vi "Create GB (2).vi"(5 "Max # of atoms":i32=9999999, 6 "Edge Duplication Range":dbl=3.0, 7 "Skip cleanup if no subset":bool=TRUE, 8 "Reduce to Repeating":T3={"Slab X"=4.6, "Slab Y"=4.0, "Tolerance (A)"=0.5, "Presorted?"=FALSE}, 9 "Min Seperation Distance (A)":dbl=2.0, 10 "Grain Growth and Geometry":T4={"Min Grain 1 Length (A)"=6.0, "Min Grain 2 Length (A)"=6.0, "Max Grain Height (A)"=90.0, "Max Grain Width (A)"=90.0, "Grain 1 Start"=-0.001, "Overlap Region (A)"=0.001}, 11 "Grain Boundary Definition":T5={"Grain 1 Orientation"=[1.0, 0.6019417241891012, 0.029651947654046266], "Grain 2 Orientation"=[1.0, 0.730727623275494, 0.2205637301176], "Twist Angle (Deg)"=0.0, "Translation Vector"=[0.0, 0.0, 0.0]}) -> (0 "GB Data":string[][](array[string])=[["Grain 1, h", "Grain 1, k", "Grain 1, L", "Grain 2, h", "Grain 2, k", "Grain 2, L", "Twist Angle (Deg)", "Translation Tx", "Translation Ty", "Translation Tz", "Tilt Angle (Deg)", "Viewing Angle, h", "Viewing Angle, k", "Viewing Angle, L", "Grain 1 Length (factor)", "Grain 2 Length (factor", "Max Grain Height (A)", "Max Grain Width (A)", "Grain 1 Start", "Overlap Region (A)", "Reduction Slab X", "Reduction Slab Y", "Reduction Tolerance (A)", "Min Atomic Separation Distance", "Edge Duplication Range", "# Atoms"], ["1.000000", "0.601942", "0.029652", "1.000000", "0.730728", "0.220564", "0.000000", "0.000000", "0.000000", "0.000000", "10.024930", "1.000000", "-1.661290", "0.000000", "1.000000", "1.000000", "90.000000", "90.000000", "-0.001000", "0.001000", "4.600000", "4.000000", "0.500000", "2.000000", "3.000000", "12135.000000"]], 1 "Reduced Orthorhombic?":bool, 2 "Reduced Rhombahedral?":bool, 3 "Grain Boundary":T6={"Structure Name"="(0.00) twist [1.000,0.602,0.030] [1.000,0.731,0.221] (0.00,0.00,0.00)T GB", "Lattice vector a"=[270.03, 0.0, 0.0], "Lattice vector b"=[0.0, 270.03, 0.0], "Lattice vector c"=[0.0, 0.0, 6.006], "Atoms Array"=[{"Atom Name"="Cd", "Positions (Direct)"=array6055x3[18165 elements], "Positions (Cartesian)"=array6055x3[18165 elements]}, {"Atom Name"="Te", "Positions (Direct)"=array6080x3[18240 elements], "Positions (Cartesian)"=array6080x3[18240 elements]}], "# of atoms"=12135} {"Atoms Array"."Positions (Cartesian)" format="%#_4f"; "Atoms Array"."Positions (Direct)" format="%#_4f"}, 4 "Ortho and Rhom":T1(array[cluster]) {"Atoms Array"."Positions (Cartesian)" format="%#_4f"; "Atoms Array"."Positions (Direct)" format="%#_4f"})   [LabVIEW 2010]
uses:
  <vilib>/Analysis/NI_AALPro.lvlib
  <vilib>/Analysis/_algsub.llb/Real Vector Norm.vi
  <vilib>/Analysis/NI_AALBase.lvlib
  <vilib>/Analysis/baseanly.llb/A x Vector.vi
  <vilib>/Analysis/baseanly.llb/Real A x B.vi
panel:
  in  "Min Wedge Thickness (A)":dbl=5.0
  out "error out":errorcluster
  out "Original # of atoms":i32=12135
  out "Expected # of Atoms":i32=166
  in  "Integer Tolerance":dbl=0.01
  in  "Predict Best Size":bool
  out "Creation Time":T2={"Time to create primitives"=0, "Time to Grow to Box"=4152, "Time to find subset"=1109, "Time to Cleanup"=1}
  in  "Headers":string[](array[string])=["Grain 1, h", "Grain 1, k", "Grain 1, L", "Grain 2, h", "Grain 2, k", "Grain 2, L", "Twist Angle (Deg)", "Translation Tx", "Translation Ty", "Translation Tz", "Tilt Angle (Deg)", "Viewing Angle, h", "Viewing Angle, k", "Viewing Angle, L", "Grain 1 Length (factor)", "Grain 2 Length (factor", "Max Grain Height (A)", "Max Grain Width (A)", "Grain 1 Start", "Overlap Region (A)", "Reduction Slab X", "Reduction Slab Y", "Reduction Tolerance (A)", "Min Atomic Separation Distance", "Edge Duplication Range", "# Atoms"]
  out "Rhombehedral Atoms":i32=12135
  out "Orthorhombic atoms":i32=12135
  out "Time to Cleanup":u32=1
  out "Time to find subset":u32=1109
  out "Time to Grow to Box":u32=4152
  out "Time to create primitives":u32
  out "Tilt Angle":dbl=10.024929742348679
  out "# of Atoms Removed":i32=28
  out "Repeating Y Length Scale":dbl=13.227303403298492
  out "Repeating X Length Scale":dbl
  out "Mutual Viewing Angle":dbl[](array[numeric])=[1.0, -1.6612903871170226, 0.0]
  in  "Conventional Unit Cell":T6={"Structure Name"="CdTe", "Lattice vector a"=[6.615785553057252, 0.0, 0.0], "Lattice vector b"=[0.0, 6.615785553057252, 0.0], "Lattice vector c"=[0.0, 0.0, 6.615785553057252], "Atoms Array"=[{"Atom Name"="Cd", "Positions (Direct)"=[[0.0, 0.0, 0.0], [0.0, 0.5, 0.5], [0.5, 0.0, 0.5], [0.5, 0.5, 0.0]], "Positions (Cartesian)"=[[0.0, 0.0, 0.0], [0.0, 3.307892776528626, 3.307892776528626], [3.307892776528626, 0.0, 3.307892776528626], [3.307892776528626, 3.307892776528626, 0.0]]}, {"Atom Name"="Te", "Positions (Direct)"=[[0.25, 0.25, 0.25], [0.75, 0.75, 0.25], [0.75, 0.25, 0.75], [0.25, 0.75, 0.75]], "Positions (Cartesian)"=[[1.653946388264313, 1.653946388264313, 1.653946388264313], [4.96183916479294, 4.96183916479294, 1.653946388264313], [4.96183916479294, 1.653946388264313, 4.96183916479294], [1.653946388264313, 4.96183916479294, 4.96183916479294]]}], "# of atoms"=8}
  # "Primitives"
  # "Grain Growth"
  # "Make into repeating cell"
  # "Remove Collisions"
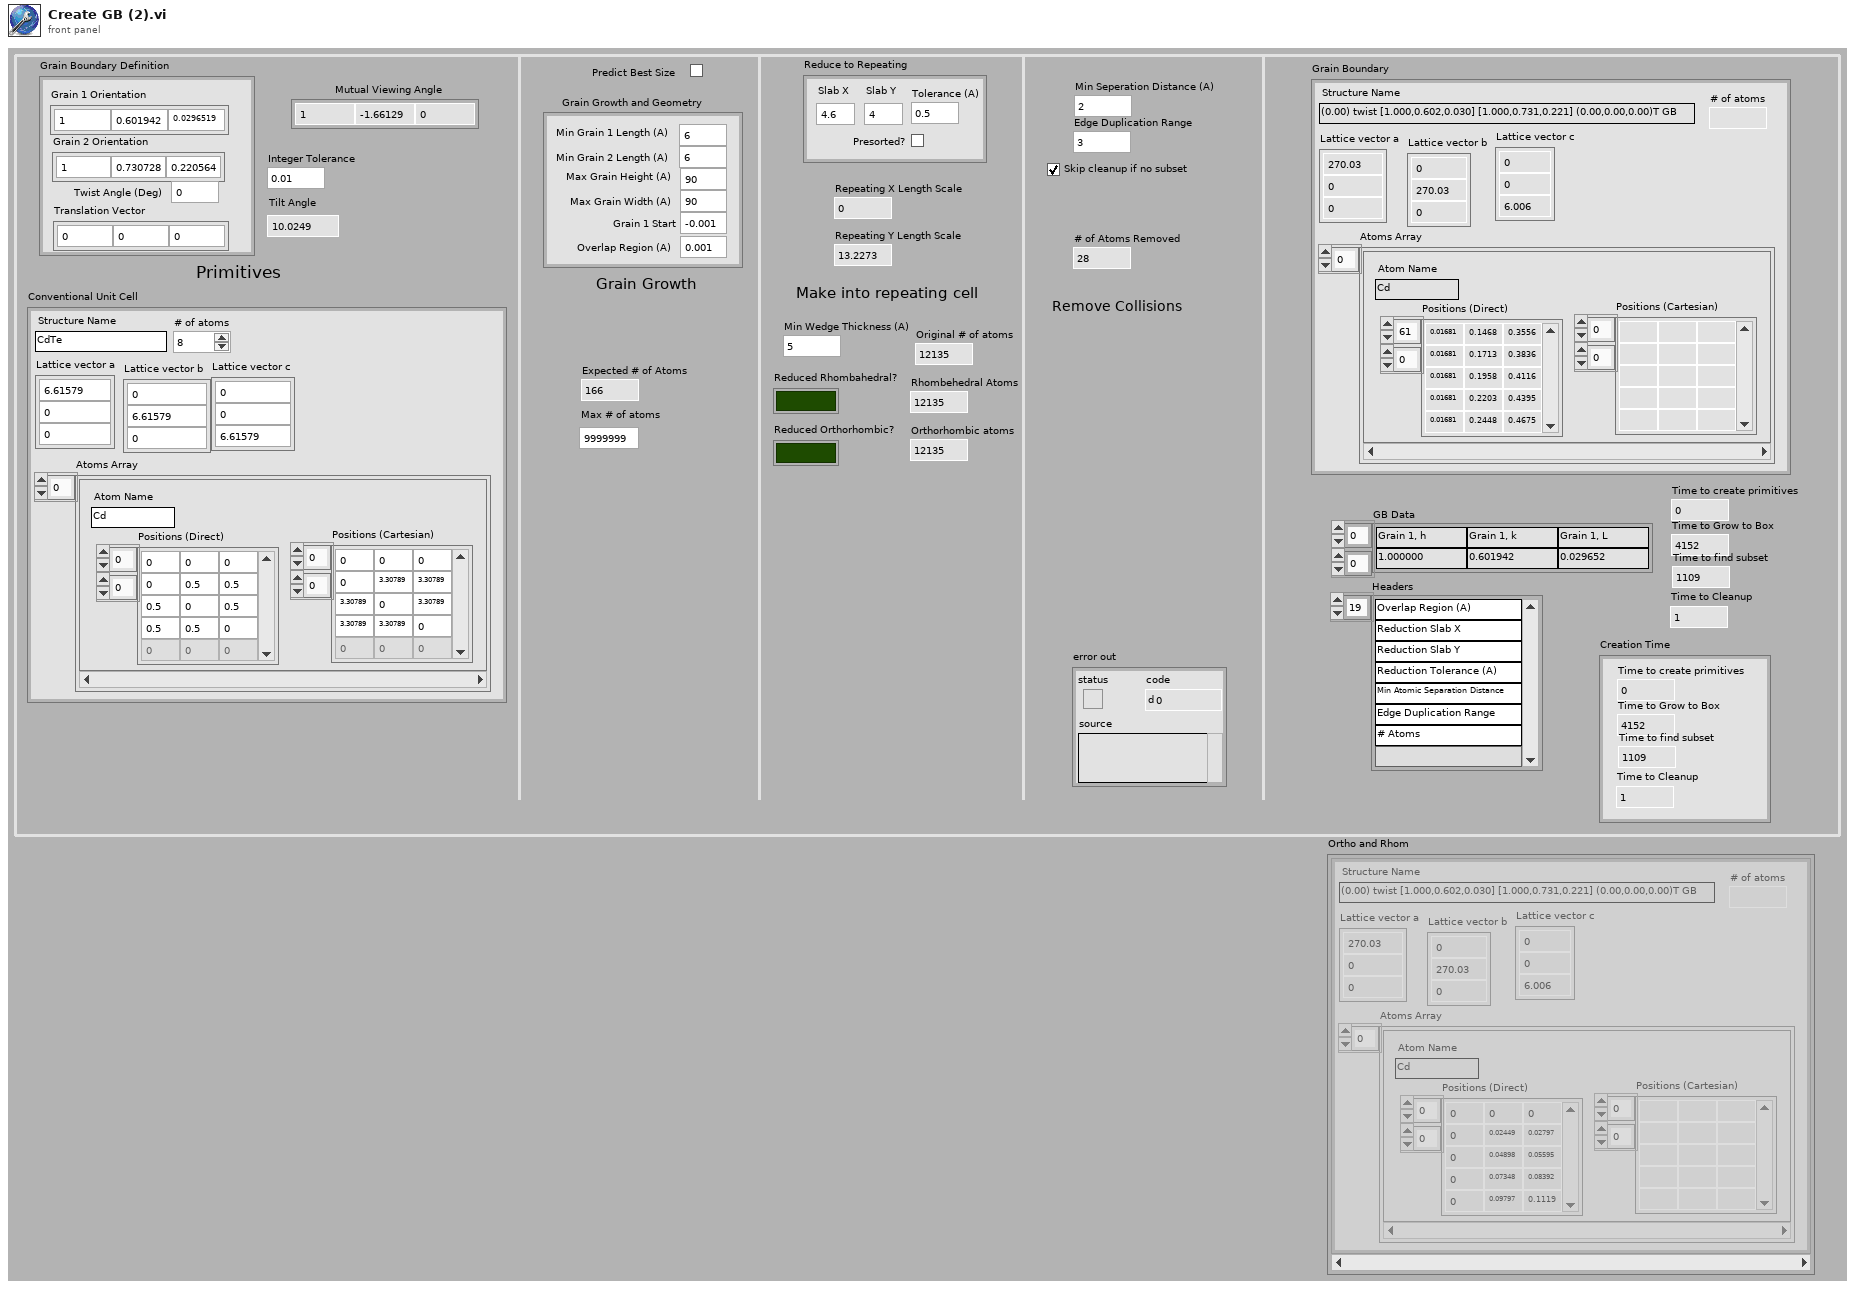
[diagram p1: front panel]
types:
  T1 = cluster{"Structure Name":string, "Lattice vector a":dbl[], "Lattice vector b":dbl[], "Lattice vector c":dbl[], "Atoms Array":cluster{"Atom Name":string, "Positions (Direct)":dbl[][], "Positions (Cartesian)":dbl[][]}[], "# of atoms":i32}[]
  T2 = cluster{"Time to create primitives":u32, "Time to Grow to Box":u32, "Time to find subset":u32, "Time to Cleanup":u32}
  T3 = cluster{"Slab X":dbl, "Slab Y":dbl, "Tolerance (A)":dbl, "Presorted?":bool}
  T4 = cluster{"Min Grain 1 Length (A)":dbl, "Min Grain 2 Length (A)":dbl, "Max Grain Height (A)":dbl, "Max Grain Width (A)":dbl, "Grain 1 Start":dbl, "Overlap Region (A)":dbl}
  T5 = cluster{"Grain 1 Orientation":dbl[], "Grain 2 Orientation":dbl[], "Twist Angle (Deg)":dbl, "Translation Vector":dbl[]}
  T6 = cluster{"Structure Name":string, "Lattice vector a":dbl[], "Lattice vector b":dbl[], "Lattice vector c":dbl[], "Atoms Array":cluster{"Atom Name":string, "Positions (Direct)":dbl[][], "Positions (Cartesian)":dbl[][]}[], "# of atoms":i32}
  T7 = cluster{"Grain 1 Orientation":dbl[], "Grain 2 Orientation":dbl[], "Twist Angle (Deg)":dbl}
  T8 = typedef "NI_Matrix.lvlib/RealMatrix.ctl" = dbl[][]
  T9 = cluster{"Z Min":dbl, "Max Grain Width (A)":dbl, "Z Min":dbl, "Max Grain Height (A)":dbl, "Grain 1 Start":dbl, "# of Atoms":i32}
  T10 = cluster{"Z Min":dbl, "Max Grain Width (A)":dbl, "Z Min":dbl, "Max Grain Height (A)":dbl, dbl, void}
  T11 = cluster{"X Min":dbl, "X Max":dbl, "Y Min":dbl, "Y Max":dbl, "Z Min":dbl, "Z Max":dbl}
  T12 = cluster{"Z Min":dbl, void, "Z Min":dbl, void, "Grain 1 Start":dbl, void}
  T13 = cluster{"Z Min":dbl, void, "Z Min":dbl, void, "Grain 1 Start":dbl, "# of Atoms":i32}
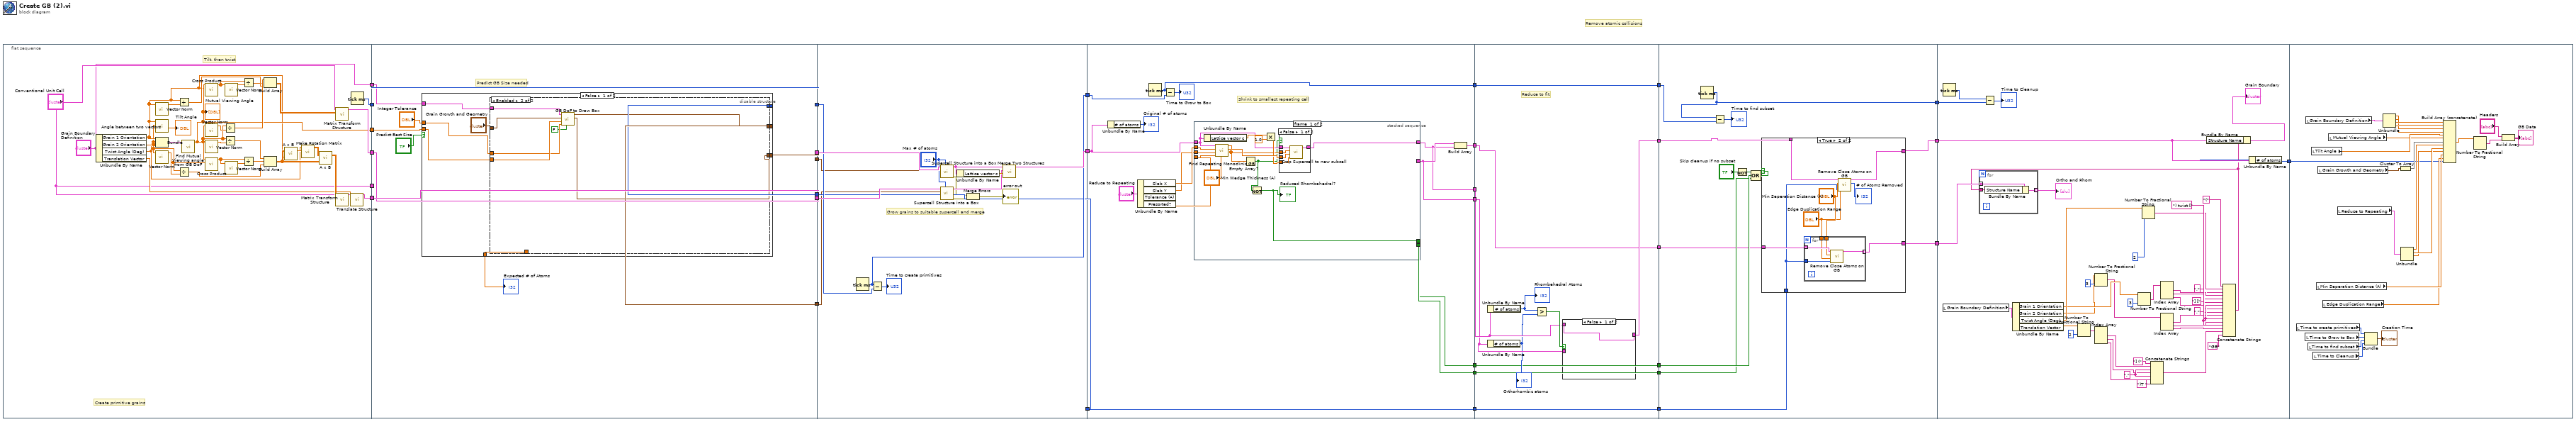
[diagram p0: block diagram]
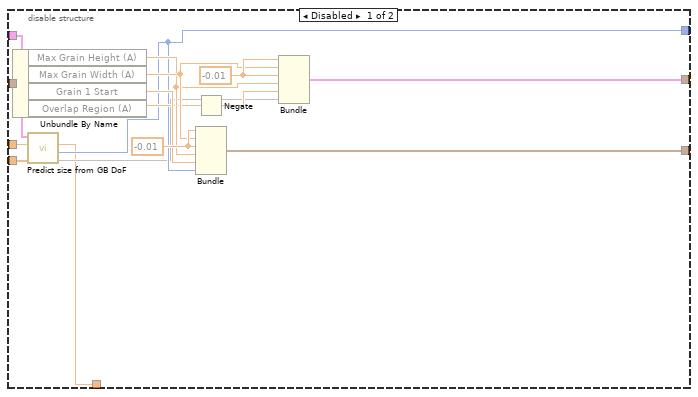
[diagram p2: hidden frame]
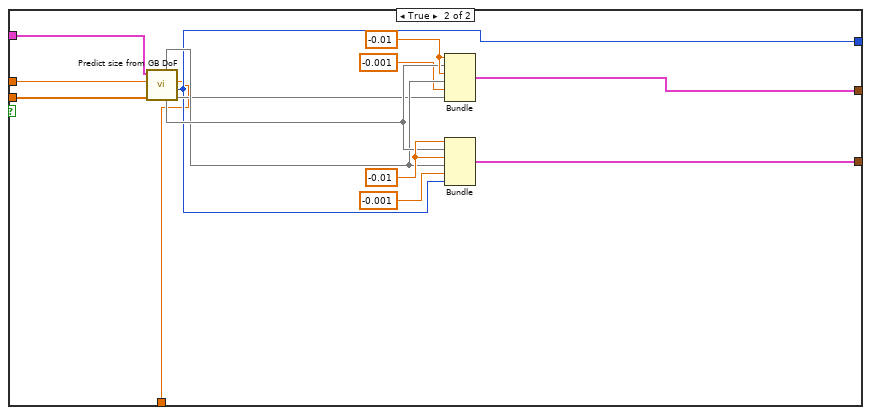
[diagram p3: hidden frame]
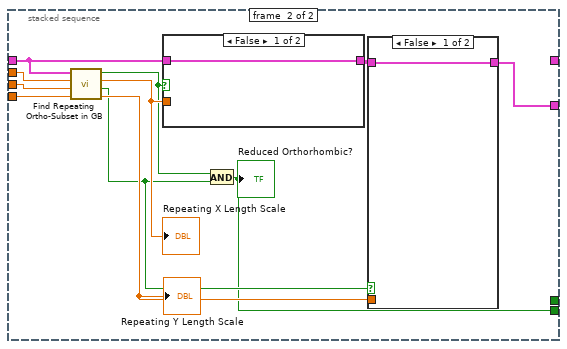
[diagram p5: hidden frame]
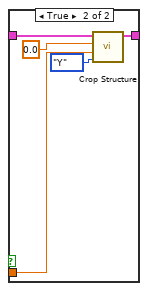
[diagram p6: hidden frame]
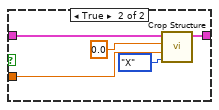
[diagram p7: hidden frame]
diagram:
  # "Remove atomic collisions"
  n1 = flat-sequence {
    tunnel: [w45] -> w15
    tunnel: [w56] -> w14
    tunnel: [w42] -> w13
    tunnel: ["Conventional Unit Cell"] -> w12
    tunnel: [w38] -> w11
    tunnel: ["Grain Boundary Definition"] -> w10
    tunnel: w15 -> [w75]
    tunnel: [w75] -> w9
    tunnel: w14 -> [w74]
    tunnel: [w74] -> w8
    tunnel: w13 -> [w73]
    tunnel: [w73] -> w7
    tunnel: w12 -> [_]
    tunnel: w11 -> [w72]
    tunnel: w10 -> [w71]
    tunnel: [w69] -> w6
    tunnel: [w68] -> w5
    tunnel: [w67] -> w4
    tunnel: w9 -> [w135]
    tunnel: w8 -> [w136]
    tunnel: [w131] -> w31
    tunnel: w7 -> [w129]
    tunnel: [w128] -> w30
    tunnel: [w127] -> w28
    tunnel: w6 -> [w122]
    tunnel: w5 -> [w121]
    tunnel: w4 -> [w127]
    tunnel: w31 -> [w143]
    tunnel: [w138] -> w27
    tunnel: w30 -> [w150]
    tunnel: [w148] -> w25
    tunnel: w28 -> [w147]
    tunnel: [w147] -> w23
    tunnel: [w139] -> w21
    tunnel: [w142] -> w19
    tunnel: [w141] -> w18
    tunnel: [w137] -> w3
    tunnel: w27 -> [w201]
    tunnel: [w199] -> w26
    tunnel: w25 -> [w204]
    tunnel: [w204] -> w24
    tunnel: w23 -> [w203]
    tunnel: [w203] -> w22
    tunnel: w21 -> [w200]
    tunnel: w19 -> [w195]
    tunnel: w18 -> [w196]
    tunnel: [w196] -> w17
    tunnel: [w195] -> w16
    tunnel: w3 -> [w194]
    tunnel: [w194] -> w2
    tunnel: w26 -> [w219]
    tunnel: [w218] -> w32
    tunnel: w24 -> [w216]
    tunnel: [w215] -> w29
    tunnel: w22 -> [w213]
    tunnel: w17 -> [w210]
    tunnel: w16 -> [w209]
    tunnel: w2 -> [w208]
    tunnel: [w207] -> w1
    tunnel: w32 -> [w248]
    tunnel: w29 -> [w249]
    tunnel: [w247] -> w20
    tunnel: w1 -> [w237]
    tunnel: w20 -> [w290]
    frame #0 {
      # "Tilt, then twist"
      # "Create primitive grains"
      n2 = Unbundle By Name("Grain Boundary Definition") -> ("Grain 1 Orientation"=w36:dbl[], "Grain 2 Orientation"=w35:dbl[], "Twist Angle (Deg)"=w34:dbl, "Translation Vector"=w43:dbl[])
      n3 = call-poly <vilib>:"Vector Norm.vi"("Input Vector"=w36) -> ("norm"=w62:dbl)  [unwired: 9 in, 1 out]
      n4 = call "Angle between two vectors.vi"("Vector 2"=w35, "Vector 1"=w36) -> ("Angle (Degrees)"=→"Tilt Angle":dbl)  [unwired: 7 in, 2 out]
      n5 = Bundle("Grain 1 Orientation"=w36, "Grain 2 Orientation"=w35, "Twist Angle (Deg)"=w34) -> (w33:T7)  [unwired: 1 in]
      n6 = call-poly <vilib>:"Vector Norm.vi"("Input Vector"=w35) -> ("norm"=w48:dbl)  [unwired: 9 in, 1 out]
      n7 = Divide(x=w36, y=w62) -> (x/y=w60:dbl[])
      n8 = Divide(x=w35, y=w48) -> (x/y=w50:dbl[])
      n9 = call "Find Mutual Viewing angle from GB DoF.vi"("Grain Boundary Macro DoF"=w33) -> ("Mutual Viewing Angle"=w38:dbl[])  [unwired: 8 in, 2 out]
      "Mutual Viewing Angle" <- w38
      n10 = call <vilib>:"Cross Product.vi"("B Vector"=w36, "A Vector"=w38) -> ("Cross Product"=w58:dbl[])  [unwired: 8 in, 1 out]
      n11 = call-poly <vilib>:"Vector Norm.vi"("Input Vector"=w38) -> ("norm"=w64:dbl)  [unwired: 9 in, 1 out]
      n12 = call-poly <vilib>:"Vector Norm.vi"("Input Vector"=w38) -> ("norm"=w46:dbl)  [unwired: 9 in, 1 out]
      n13 = call <vilib>:"Cross Product.vi"("B Vector"=w35, "A Vector"=w38) -> ("Cross Product"=w51:dbl[])  [unwired: 8 in, 1 out]
      n14 = Divide(x=w38, y=w64) -> (x/y=w61:dbl[])
      n15 = Divide(x=w38, y=w46) -> (x/y=w49:dbl[])
      n16 = call-poly <vilib>:"Vector Norm.vi"("Input Vector"=w58) -> ("norm"=w63:dbl)  [unwired: 9 in, 1 out]
      n17 = call-poly <vilib>:"Vector Norm.vi"("Input Vector"=w51) -> ("norm"=w47:dbl)  [unwired: 9 in, 1 out]
      n18 = Divide(x=w58, y=w63) -> (x/y=w57:dbl[])
      n19 = Divide(x=w51, y=w47) -> (x/y=w55:dbl[])
      n20 = Build Array(w61, w57, w60) -> (w59:T8)
      n21 = Build Array(w49, w55, w50) -> (w40:T8)
      n22 = call-poly <vilib>:"A x B.vi"("Vector"=w36, "A"=w40) -> ("A x Vector"=w39:dbl[])  [unwired: 1 out]
      n23 = call "Make Rotation Matrix.vi"("Rotation Axis"=w39, "Rotation Angle (Degree)"=w34) -> ("Rotation Matrix"=w53:T8)  [unwired: 9 in]
      n24 = call-poly <vilib>:"A x B.vi"("B"=w40, "A"=w53) -> ("A x B"=w52:T8)  [unwired: 1 out]
      n25 = call "Matrix Transform Structure.vi"("Matrix Transform"=w59, "Original Structure"="Conventional Unit Cell") -> ("After Transform"=w56:T6)  [unwired: 9 in]
      n26 = call "Matrix Transform Structure.vi"("Matrix Transform"=w52, "Original Structure"="Conventional Unit Cell") -> ("After Transform"=w54:T6)  [unwired: 9 in]
      n27 = call "Translate Structure.vi"("Translation Vector (Cartesian)"=w43, "Atomic Structure"=w54) -> ("Shifted Structure"=w45:T6)  [unwired: 9 in]
      n28 = Tick Count (ms)() -> (millisecond timer value=w42:u32)
    }
    frame #1 {
      # "Predict GB Size needed"
      n29 = case shown="False" "Predict Best Size" {
        tunnel: w72 -> [w80 w120]
        tunnel: w71 -> [w77 w119]
        tunnel: [w82 w116] -> w69
        tunnel: [w81 w110] -> w68
        tunnel: [w79 w109] -> w67
        tunnel: "Integer Tolerance" -> [w76 w108]
        tunnel: [w78 w107] -> w65
        frame False {
          n30 = disable-structure shown="Enabled" {
            disable-tunnel: "Grain Growth and Geometry" -> [w99 w106]
            disable-tunnel: [w96 w100] -> w82
            disable-tunnel: [w90 w101] -> w81
            disable-tunnel: w80 -> [w89 w104]
            disable-tunnel: [w88 _] -> w79
            disable-tunnel: [w86 _] -> w78
            disable-tunnel: w77 -> [w85 w105]
            disable-tunnel: w76 -> [w84 w103]
            frame Disabled {
              w95 = -0.01 ("Z Min")
              w98 = -0.01 ("Z Min")
              n31 = Unbundle By Name(w99) -> ("Max Grain Height (A)"=w93:dbl, "Max Grain Width (A)"=w94:dbl, "Grain 1 Start"=w97:dbl, "Overlap Region (A)"=w92:dbl)
              n32 = call "Predict size from GB DoF.vi"("Integer Tolerance"=w89, "Mutual Viewing Angle"=w84, "Grain Boundary Definition"=w85) -> (0:w87, "# of Atoms"=w88:i32, "Expected Volume (A3)"=w86:dbl)  [unwired: 5 in, 1 out]
              n33 = Negate(x=w92) -> (-x=w91:dbl)
              n34 = Bundle("Z Min"=w98, "Max Grain Width (A)"=w94, "Z Min"=w98, "Max Grain Height (A)"=w93, "Grain 1 Start"=w97, "# of Atoms"=w88) -> (w96:T9)  [unwired: 1 in]
              n35 = Bundle("Z Min"=w95, "Max Grain Width (A)"=w94, "Z Min"=w95, "Max Grain Height (A)"=w93, w91, w87) -> (w90:T10)  [unwired: 1 in]
            }
            frame Enabled {
              n36 = call "GB DoF to Draw Box.vi"("Force Size to Min"=FALSE, "Integer Tolerance"=w103, "Mutual Viewing Angle"=w104, "Grain Growth and Geometry"=w106, "Grain Boundary Definition"=w105) -> ("Draw Box Grain 2"=w100:T11, "Draw Box Grain 1"=w101:T11)  [unwired: 5 in]
            }
          }
        }
        frame True {
          w115 = -0.01 ("Z Min")
          w118 = -0.01 ("Z Min")
          n37 = call "Predict size from GB DoF.vi"("Integer Tolerance"=w120, "Mutual Viewing Angle"=w108, "Grain Boundary Definition"=w119) -> (0:w111, "# of Atoms"=w109:i32, "Expected Volume (A3)"=w107:dbl, 4:w114, 5:w113)  [unwired: 3 in, 1 out]
          n38 = Bundle("Z Min"=w115, w114, "Z Min"=w115, w113, "Grain 1 Start"=-0.001, w111) -> (w110:T12)  [unwired: 1 in]
          n39 = Bundle("Z Min"=w118, w114, "Z Min"=w118, w113, "Grain 1 Start"=-0.001, "# of Atoms"=w109) -> (w116:T13)  [unwired: 1 in]
        }
      }
      "Expected # of Atoms" <- w65
    }
    frame #2 {
      # "Grow grains to suitable supercell and merge"
      n40 = Tick Count (ms)() -> (millisecond timer value=w128:u32)
      n41 = Subtract(x=w128, y=w129) -> (x-y=→"Time to create primitives":u32)
      n42 = call "Supercell Structure into a Box.vi"("Max # of atoms"="Max # of atoms", "Draw Box"=w122, "Subcrystal"=w136) -> ("error out"=w125:errorcluster, "Expanded cubic Structure"=w132:T6)  [unwired: 6 in, 1 out]
      n43 = call "Supercell Structure into a Box.vi"("Max # of atoms"="Max # of atoms", "Draw Box"=w121, "Subcrystal"=w135) -> ("error out"=w124:errorcluster, "Expanded cubic Structure"=w133:T6)  [unwired: 6 in, 1 out]
      n44 = Unbundle By Name(w132) -> ("Lattice vector c"=w134:dbl[])
      n45 = Merge Errors(w125, w124) -> (→"error out":errorcluster)
      n46 = call "Merge Two Structures.vi"("Translation Vector (1 to 2)"=w134, "Atomic Structure 2"=w133, "Atomic Structure 1"=w132) -> ("Atomic Structure of 1 + 2 by T"=w131:T6)  [unwired: 8 in]
    }
    frame #3 {
      # "Shrink to smallest repeating cell"
      n47 = Unbundle By Name(w143) -> ("# of atoms"=→"Original # of atoms":i32)
      n48 = Unbundle By Name("Reduce to Repeating") -> ("Slab X"=w146:dbl, "Slab Y"=w145:dbl, "Tolerance (A)"=w144:dbl)  [unwired: 1 out]
      n49 = Tick Count (ms)() -> (millisecond timer value=w148:u32)
      n50 = Subtract(x=w148, y=w150) -> (x-y=→"Time to Grow to Box":u32)
      n51 = stacked-sequence {
        tunnel: [w153 _] -> w138
        tunnel: w146 -> [w159 w181]
        tunnel: w145 -> [w158 w180]
        tunnel: w144 -> [w157 w179]
        tunnel: w143 -> [w160 w178]
        tunnel: [_ w171] -> w139
        tunnel: [_ w172] -> w142
        tunnel: [w154 _] -> w141
        frame #0 {
          n52 = Unbundle By Name(w160) -> ("Lattice vector c"=w162:dbl[])
          n53 = call "Find Repeating Monoclinic GB.vi"("Min Wedge Thickness (A)"="Min Wedge Thickness (A)", "Tolerance (A)"=w157, "Slab Y"=w158, "Slab X"=w159, "Supercell Structure"=w160) -> ("New Lattice Vector b"=w164:dbl[], "New Lattice Vector a"=w156:dbl[])  [unwired: 4 in, 1 out]
          n54 = Empty Array?(array=w156) -> (empty?=w155:bool)
          n55 = Not(x=w155) -> (.not. x?=w154:bool)
          "Reduced Rhombahedral?" <- w154
          n56 = Multiply(x=w162, y=1.0) -> (x*y=w161:dbl[])
          n57 = case shown="False" w155 {
            tunnel: w164 -> [w169 _]
            tunnel: w156 -> [w168 _]
            tunnel: w161 -> [w167 _]
            tunnel: w160 -> [w166 w170]
            tunnel: [w165 w170] -> w153
            frame False {
              n58 = call "Crop Supercell to new subcell.vi"("New Lattice Vector c"=w167, "New Lattice Vector b"=w169, "New Lattice Vector a"=w168, "Supercell Structure"=w166) -> ("Reduced Structure"=w165:T6)  [unwired: 7 in]
            }
            frame True {
            }
          }
        }
        frame #1 {
          n59 = call "Find Repeating Ortho-Subset in GB.vi"("Tolerance (A)"=w179, "Slab Y"=w180, "Slab X"=w181, "Grain Boundary"=w178) -> ("Repeating Y Length Scale"=w175:dbl, "Subset Y found?!"=w173:bool, "Repeating X Length Scale"=w176:dbl, "Subset X found?!"=w174:bool)  [unwired: 4 in]
          "Repeating X Length Scale" <- w176
          "Repeating Y Length Scale" <- w175
          n60 = case shown="False" w174 {
            tunnel: w178 -> [w188 w193]
            tunnel: [w188 w190] -> w177
            tunnel: w176 -> [_ w189]
            frame False {
            }
            frame True {
              n61 = call "Crop Structure.vi"("Cropping Index"=enum16{"X", "Y", "Z"}."X", "Upper Bound Z"=w189, "Lower bound Z"=0.0, "Input Structure"=w193) -> ("Cropped Structure"=w190:T6)  [unwired: 7 in]
            }
          }
          n62 = And(x=w174, y=w173) -> (x .and. y?=w172:bool)
          "Reduced Orthorhombic?" <- w172
          n63 = case shown="False" w173 {
            tunnel: w177 -> [w182 w187]
            tunnel: w175 -> [_ w185]
            tunnel: [w182 w183] -> w171
            frame False {
            }
            frame True {
              n64 = call "Crop Structure.vi"("Cropping Index"=enum16{"X", "Y", "Z"}."Y", "Upper Bound Z"=w185, "Lower bound Z"=0.0, "Input Structure"=w187) -> ("Cropped Structure"=w183:T6)  [unwired: 7 in]
            }
          }
        }
      }
      n65 = Build Array(w139, w138) -> (w137:T1)
    }
    frame #4 {
      # "Reduce to fit"
      n66 = Unbundle By Name(w200) -> ("# of atoms"=w197:i32)
      "Orthorhombic atoms" <- w197
      n67 = Unbundle By Name(w201) -> ("# of atoms"=w198:i32)
      "Rhombehedral Atoms" <- w198
      n68 = Greater?(x=w198, y=w197) -> (0:w202:bool)
      n69 = case shown="False" w202 {
        tunnel: [w205 w206] -> w199
        tunnel: w201 -> [w205 _]
        tunnel: w200 -> [_ w206]
        frame False {
        }
        frame True {
        }
      }
    }
    frame #5 {
      n70 = Tick Count (ms)() -> (millisecond timer value=w215:u32)
      n71 = Subtract(x=w215, y=w216) -> (x-y=→"Time to find subset":u32)
      n72 = Not(x="Skip cleanup if no subset") -> (.not. x?=w212:bool)
      n73 = Compound Arithmetic op=OR(w212, w210, w209) -> (w211:bool)
      n74 = case shown="True" w211 {
        tunnel: w219 -> [w221 w228]
        tunnel: [w221 w227] -> w218
        tunnel: w213 -> [_ w223]
        tunnel: w208 -> [w220 w226]
        tunnel: [w220 w222] -> w207
        frame False {
        }
        frame True {
          n75 = for {
            tunnel: w226 -> [w234] mode=indexing
            tunnel: [w233] -> w222 mode=indexing
            tunnel: "Min Seperation Distance (A)" -> [w232]
            tunnel: "Edge Duplication Range" -> [w231]
            tunnel: w223 -> [w230]
            n76 = call "Remove Close Atoms on GB.vi"("Grain Boundary Location (A)"=w230, "Edge Duplication Range"=w231, "Minimally Allowable Distance (A)"=w232, "Structure"=w234) -> ("Structure with atoms removed"=w233:T6)  [unwired: 6 in, 1 out]
          }
          n77 = call "Remove Close Atoms on GB.vi"("Grain Boundary Location (A)"=w223, "Edge Duplication Range"="Edge Duplication Range", "Minimally Allowable Distance (A)"="Min Seperation Distance (A)", "Structure"=w228) -> ("# of Atoms Removed"=→"# of Atoms Removed":i32, "Structure with atoms removed"=w227:T6)  [unwired: 6 in]
        }
      }
    }
    frame #6 {
      w270 = "," ("string")
      w263 = "," ("string")
      n78 = local read "Grain Boundary Definition"() -> (w273:T5)
      n79 = Tick Count (ms)() -> (millisecond timer value=w250:u32)
      n80 = Subtract(x=w250, y=w249) -> (x-y=→"Time to Cleanup":u32)
      n81 = Unbundle By Name(w273) -> ("Grain 1 Orientation"=w244:dbl[], "Grain 2 Orientation"=w241:dbl[], "Twist Angle (Deg)"=w274:dbl, "Translation Vector"=w275:dbl[])
      n82 = Number To Fractional String(number=w275, precision (6)=i16 2) -> (F-format string=w266:string[])  [unwired: 2 in]
      n83 = Number To Fractional String(number=w241, precision (6)=i16 3) -> (F-format string=w240:string[])  [unwired: 2 in]
      n84 = Index Array(array=w266) -> (element #1=w267:string, element #2=w269:string, element #3=w271:string)  [unwired: 3 in]
      n85 = Number To Fractional String(number=w244, precision (6)=i16 3) -> (F-format string=w243:string[])  [unwired: 2 in]
      n86 = Number To Fractional String(number=w274, precision (6)=i16 2) -> (F-format string=w254:string)  [unwired: 2 in]
      n87 = Concatenate Strings("] (" ("string"), w267, w270, w269, w270, w271, ")T " ("string")) -> (w239:string)
      n88 = Index Array(array=w243) -> (element #1=w256:string, element #2=w258:string, element #3=w259:string)  [unwired: 3 in]
      n89 = Index Array(array=w240) -> (element #1=w261:string, element #2=w262:string, element #3=w264:string)  [unwired: 3 in]
      n90 = Concatenate Strings("(" ("string"), w254, ") twist [" ("string"), w256, "," ("string"), w258, w263, w259, "] [" ("string"), w261, w263, w262, w263, w264, w239, "GB" ("string")) -> (w236:string)
      n91 = for {
        tunnel: w237 -> [w278] mode=indexing
        tunnel: w236 -> [w277]
        tunnel: [w276] -> w235 mode=indexing
        n92 = Bundle By Name(cluster=w278, "Structure Name"=w277) -> (w276:T6)
      }
      "Ortho and Rhom" <- w235
      n93 = Bundle By Name(cluster=w248, "Structure Name"=w236) -> (→"Grain Boundary":T6)
      n94 = Unbundle By Name(w248) -> ("# of atoms"=w247:i32)
    }
    frame #7 {
      n95 = local read "Time to create primitives"() -> (w282:u32)
      n96 = local read "Time to Grow to Box"() -> (w281:u32)
      n97 = local read "Grain Boundary Definition"() -> (w303:T5)
      n98 = local read "Time to find subset"() -> (w280:u32)
      n99 = local read "Tilt Angle"() -> (w286:dbl)
      n100 = local read "Time to Cleanup"() -> (w283:u32)
      n101 = local read "Min Seperation Distance (A)"() -> (w292:dbl)
      n102 = local read "Grain Growth and Geometry"() -> (w298:T4)
      n103 = local read "Edge Duplication Range"() -> (w291:dbl)
      n104 = local read "Mutual Viewing Angle"() -> (w285:dbl[])
      n105 = local read "Reduce to Repeating"() -> (w296:T3)
      n106 = Bundle("Time to create primitives"=w282, "Time to Grow to Box"=w281, "Time to find subset"=w280, "Time to Cleanup"=w283) -> (→"Creation Time":T2)  [unwired: 1 in]
      n107 = Unbundle(w303) -> ("Grain 1 Orientation"=w302:dbl[], "Grain 2 Orientation"=w301:dbl[], "Twist Angle (Deg)"=w300:dbl, "Translation Vector"=w299:dbl[])
      n108 = Cluster To Array(cluster=w298) -> (array=w297:dbl[])
      n109 = Unbundle(w296) -> ("Slab X"=w295:dbl, "Slab Y"=w294:dbl, "Tolerance (A)"=w293:dbl)  [unwired: 1 out]
      n110 = Build Array (concatenate)(w302, w301, w300, w299, w286, w285, w297, w295, w294, w293, w292, w291, w290) -> (w289:dbl[])
      n111 = Number To Fractional String(number=w289) -> (F-format string=w288:string[])  [unwired: 3 in]
      n112 = Build Array("Headers", w288) -> (→"GB Data":string[][])
    }
  }
